vi "ABC Get Last Position.vi"(1 "Response":string) -> (2 "Position":dbl)   [LabVIEW 2020]
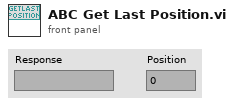
[diagram p1: front panel]
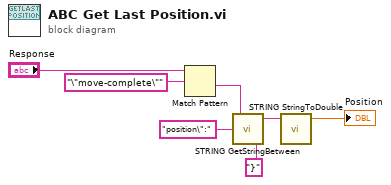
[diagram p0: block diagram]
diagram:
  n1 = Match Pattern(string="Response", regular expression="\"move-complete\"") -> (after substring=w6:string)  [unwired: 1 in, 3 out]
  n2 = call <userlib>:"STRING GetStringBetween.vi"("EndStr"="}", "BeginStr"="position\":", "StrIn"=w6) -> ("StrOut"=w3:string)  [unwired: 2 in]
  n3 = call <userlib>:"STRING StringToDouble.vi"("DblStr"=w3) -> ("Num"=→"Position":dbl)  [unwired: 4 in]
